vi "Plugin - Acquire Meta Data.vi"(11 "Message Queues in":T2) -> ()   [LabVIEW 2019]
uses:
  support/Copy of Message Queue/All Message Queues.ctl
  support/Copy of Message Queue/Message Cluster.ctl
  support/Message Queue/Message Queue.lvlib
  support/Copy of Message Queue/Copy of Message Queue.lvlib
panel:
  in  "MetaData":T1={"Operator Name"=enum."Operator Name", "Location"=enum."Location", "Sensor SN"="Sensor SN", "Cal Tube SN"="Cal Tube SN", "Comments"="Comments"}
  in  "error in":errorcluster
  out "error out":errorcluster
  in  "Next":bool
  in  "Exit":bool
  # "Enter Sensor Meta Data"
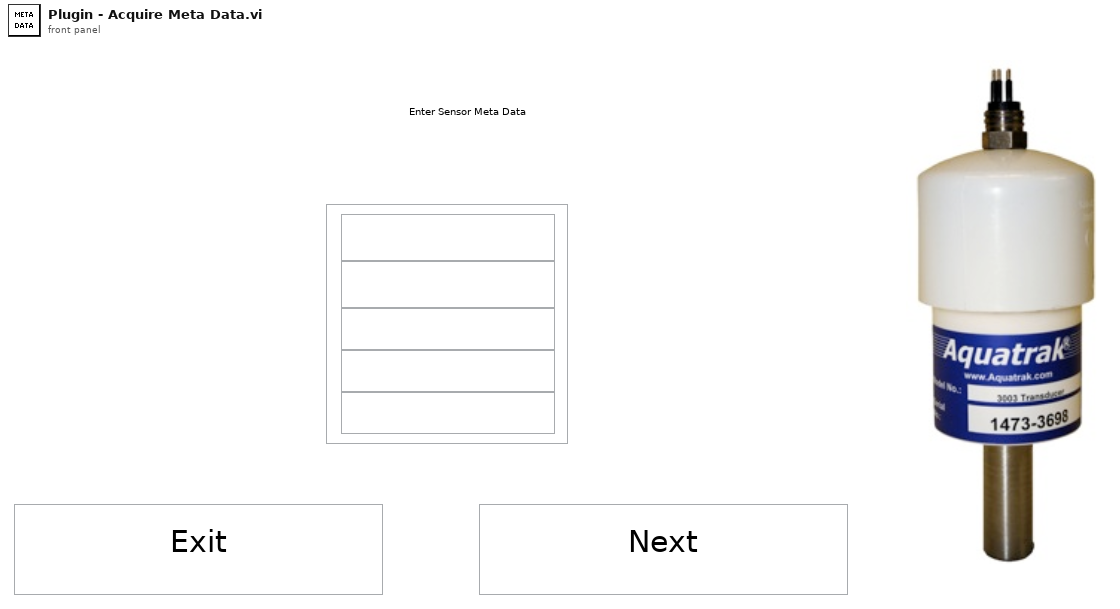
[diagram p1: front panel]
types:
  T1 = cluster{"Operator Name":enum16{"Operator Name", "Shaena", "Mark"}, "Location":enum16{"Location", "Chesapeake", "Silver Spring", "Seattle"}, "Sensor SN":string, "Cal Tube SN":string, "Comments":string}
  T2 = typedef "Copy of Message Queue.lvlib/All Message Queues.ctl" = cluster{"UI":refnum<queue>, "Acquisition":refnum<queue>, "Logging":refnum<queue>, "Analyze":refnum<queue>}
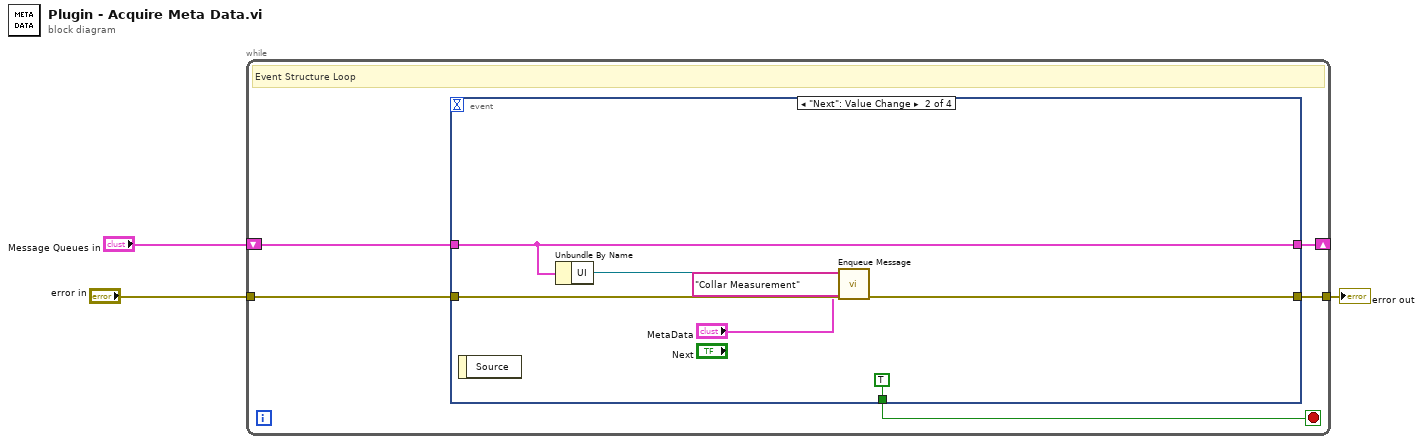
[diagram p0: block diagram]
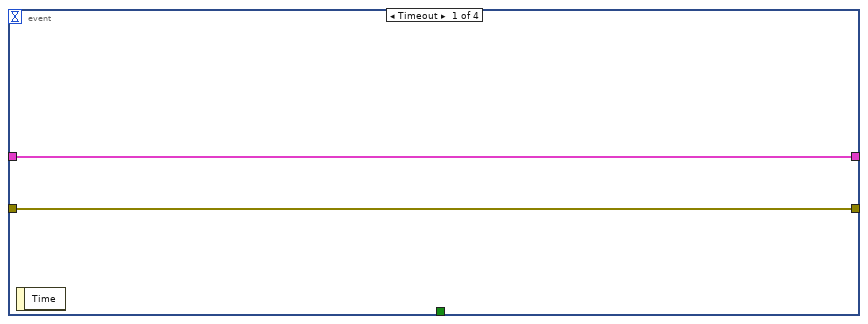
[diagram p2: hidden frame]
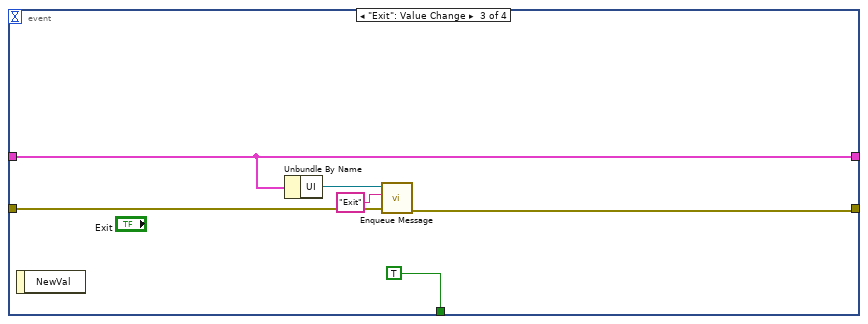
[diagram p3: hidden frame]
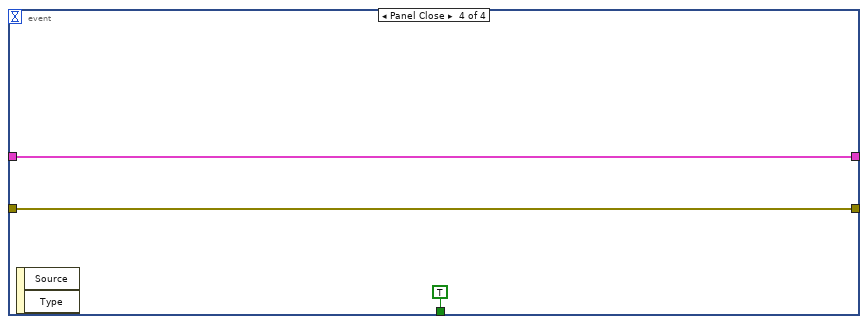
[diagram p4: hidden frame]
diagram:
  n1 = while {
    shift-right: [w7] -> _
    shift-left: "Message Queues in" -> [w6]
    tunnel: [w5] -> w2
    tunnel: "error in" -> [w4]
    stop <- w8 stop-if-true
    # "Event Structure Loop"
    n2 = event shown="[1] \"Next\": Value Change" {
      selector: _ -> [_ _ _ _]
      dyn-events: _ -> [_ _ _ _]
      timeout: _ -> [_ _ _ _]
      tunnel: [_ TRUE ("NewVal") TRUE ("NewVal") TRUE ("NewVal")] -> w8
      tunnel: w6 -> [w10 w17 w20 w26]
      tunnel: [w10 w17 w20 w26] -> w7
      tunnel: [w9 w13 w18 w24] -> w5
      tunnel: w4 -> [w9 w12 w19 w24]
      event Timeout {
        n3 = event-data() -> ()  [unwired: 1 in, 1 out]
      }
      event "Next": Value Change {
        n4 = event-data() -> ()  [unwired: 1 in, 1 out]
        n5 = Unbundle By Name(w17) -> ("UI"=w15:refnum<queue>)
        n6 = call "Enqueue Message.vi"("error in (no error)"=w12, "Message Data"="MetaData", "Message"="Collar Measurement", "Message Queue"=w15) -> ("error out"=w13:errorcluster)  [unwired: 6 in, 1 out]
      }
      event "Exit": Value Change {
        n7 = event-data() -> ()  [unwired: 1 in, 1 out]
        n8 = Unbundle By Name(w20) -> ("UI"=w21:refnum<queue>)
        n9 = call "Enqueue Message.vi"("error in (no error)"=w19, "Message"="Exit", "Message Queue"=w21) -> ("error out"=w18:errorcluster)  [unwired: 7 in, 1 out]
      }
      event Panel Close {
        n10 = event-data() -> ()  [unwired: 1 in, 2 out]
      }
    }
  }
  "error out" <- w2
